vi "Read Strings from File.vi"(8 "Error In":errorcluster, 9 "Section Name":string, 11 "Path":path) -> (0 "Error Out":errorcluster, 1 "Found?":bool, 3 "Variant Database":variant)   [LabVIEW 2020]
doc: "This VI was created for use with the Read/Write Cluster VIs. It reads all the keys and their values from the specified section and puts them in two string arrays.\n\nFreeware from Moore Good Ideas, www.mooregoodideas.com. Do not remove this line."
uses:
  Suppress Error Code - Scalar.vi
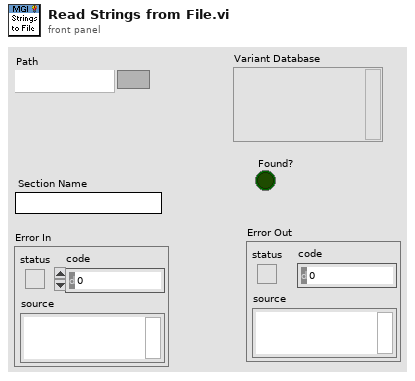
[diagram p1: front panel]
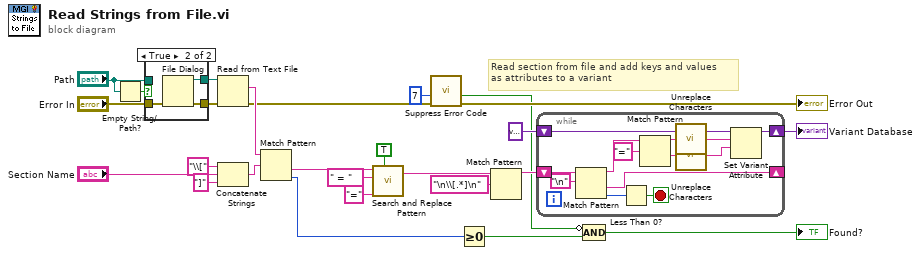
[diagram p0: block diagram]
diagram:
  # "Read section from file and add keys and values\nas attributes to a variant"
  n1 = Empty String/Path?(string/path="Path") -> (empty?=w9:bool)
  n2 = case shown="True" w9 {
    tunnel: "Error In" -> [w27 w31]
    tunnel: [w27 w30] -> w10
    tunnel: [w28 w29] -> w12
    tunnel: "Path" -> [w28 _]
    frame False {
    }
    frame True {
      n3 = File Dialog(8:w31) -> (0:w30:errorcluster, 3:w29:path)  [unwired: 6 in, 2 out]
    }
  }
  n4 = Read from Text File(file (use dialog)=w12, error in=w10) -> (text=w22:string, error out=w18:errorcluster)  [unwired: 2 in, 2 out]
  n5 = Concatenate Strings("\\[" ("string"), "Section Name", "]" ("string")) -> (w23:string)
  n6 = Match Pattern(string=w22, regular expression=w23) -> (after substring=w5:string, offset past match=w19:i32)  [unwired: 1 in, 2 out]
  n7 = call <vilib>:"Search and Replace Pattern.vi"("string"=w5, "regular expression (\"\")"=" = " ("regular expression (\"\")"), "replace string (\"\")"="=" ("replace string (\"\")"), "replace all? (F)"=TRUE) -> ("result string"=w4:string)  [unwired: 1 in, 1 out]
  n8 = call-poly "Suppress Error Code.vi"("Error In"=w18, "Error Code"=7) -> ("Error Out"=→"Error Out":errorcluster, "Error Supressed?"=w7:bool)  [unwired: 8 in]
  n9 = Greater Or Equal To 0?(x=w19) -> (x >= 0?=w6:bool)
  n10 = Match Pattern(string=w4, regular expression="\n\\[.*]\n") -> (before substring=w20:string)  [unwired: 1 in, 3 out]
  n11 = while {
    shift-right: [w42] -> _
    shift-left: w20 -> [w44]
    shift-right: [w37] -> w13
    shift-left: variant ("variant") -> [w38]
    stop <- w40 stop-if-true
    n12 = Match Pattern(string=w44, regular expression="\n") -> (before substring=w36:string, after substring=w42:string, offset past match=w41:i32)  [unwired: 1 in, 1 out]
    n13 = Less Than 0?(x=w41) -> (x < 0?=w40:bool)
    n14 = Match Pattern(string=w36, regular expression="=") -> (before substring=w35:string, after substring=w34:string)  [unwired: 1 in, 2 out]
    n15 = call "Unreplace Characters.vi"("String In"=w35) -> ("String Out"=w32:string)  [unwired: 1 in]
    n16 = call "Unreplace Characters.vi"("String In"=w34) -> ("String Out"=w33:string)  [unwired: 1 in]
    n17 = Set Variant Attribute(Variant=w38, name=w32, value=w33) -> (Variant out=w37:variant)  [unwired: 1 in, 2 out]
  }
  "Variant Database" <- w13
  n18 = Compound Arithmetic op=AND(invert w7, w6) -> (→"Found?":bool)
